vi "GetParam.vi"(8 "error in (no error)":errorcluster caption="entrée d'erreur (pas d'erreur)", 11 "Swiss_Roll.lvclass":refnum<class "Swiss_Roll.lvclass">) -> (0 "error out":errorcluster caption="sortie d'erreur", 2 "make_swiss_roll":T1={"n_samples"=100, "noise"=0.0, "random_state"=-1, "Returns"="X"} {"random_state" min=-1; "n_samples" min=1}, 3 "Swiss_Roll.lvclass":refnum<class "Swiss_Roll.lvclass">)   [LabVIEW 2020, in "Swiss_Roll.lvclass"]
doc: "Get Parameters"
uses:
  Swiss_Roll.lvclass
  Swiss_Roll.lvclass/Swiss_Roll.ctl
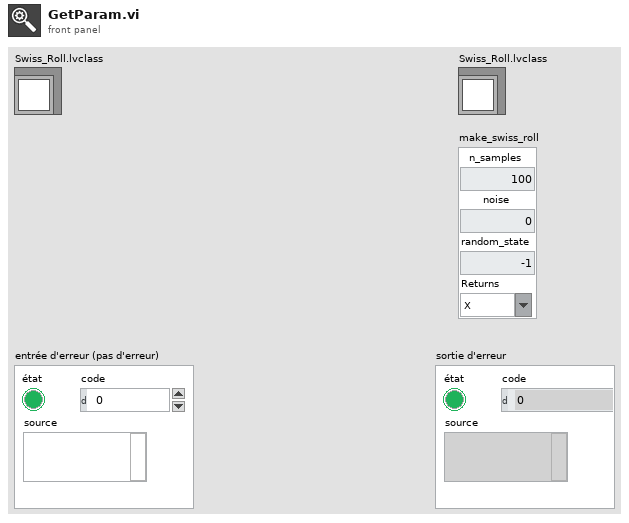
[diagram p1: front panel]
types:
  T1 = cluster{"n_samples":u32, "noise":dbl, "random_state":i32, "Returns":string}
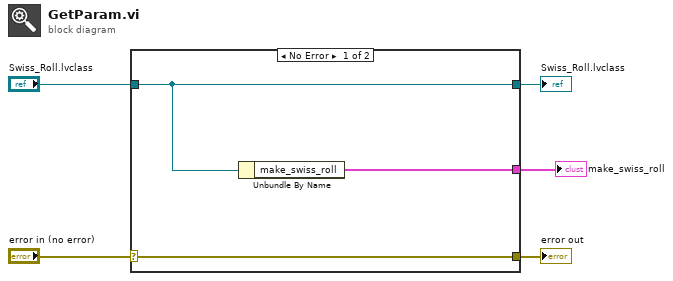
[diagram p0: block diagram]
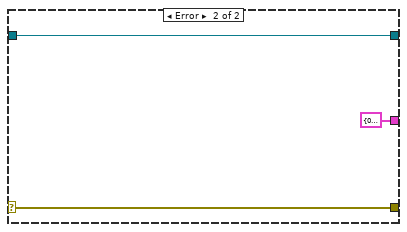
[diagram p2: hidden frame]
diagram:
  n1 = case shown="No Error" "error in (no error)" {
    selector: "error in (no error)" -> [w8 w10]
    tunnel: [w8 w10] -> w4
    tunnel: [w7 w11] -> w2
    tunnel: "Swiss_Roll.lvclass" -> [w7 w11]
    tunnel: [w6 T1 {"n_samples"=0, "noise"=0.0, "random_state"=0, "Returns"=""} ("make_swiss_roll")] -> w1
    frame No Error {
      n2 = Unbundle By Name(w7) -> ("make_swiss_roll"=w6:T1)
    }
    frame Error {
    }
  }
  "error out" <- w4
  "Swiss_Roll.lvclass" <- w2
  "make_swiss_roll" <- w1
